vi "Get Mecanum Wheel Information.vi"(8 "error in (no error)":errorcluster, 11 "wheel in":refnum<class "NI_Robotics_Wheel.lvclass">) -> (0 "error out":errorcluster, 1 "wheel name":string, 2 "wheel parameters":T1={"wheel radius"=1.0, "gear ratio"=1.0, "forward rotation direction"=0} {"forward rotation direction" items=["Clockwise", "Counterclockwise"]}, 3 "wheel out":refnum<class "NI_Robotics_Wheel.lvclass">, 4 "motor communication":refnum<class "NI_Robotics_Motor Communication.lvclass">, 5 "roller orientation":T3 items=["Left", "Right"])   [LabVIEW 2017, in "NI_Robotics_Wheel.lvclass"]
doc: "Returns information, such as <B>wheel radius</B> and <B>gear ratio</B>, for the wheel you specify. You must manually select the polymorphic instance to use."
uses:
  <vilib>/robotics/Steering/Wheel/NI_Robotics_Wheel.lvclass
  <vilib>/robotics/Steering/Mecanum Wheel/Roller Orientation.ctl
  <vilib>/robotics/Steering/Wheel/Wheel Parameters.ctl
  <vilib>/robotics/Steering/Wheel/Rotation Direction.ctl
  <vilib>/robotics/Actuation/Motor Communication/NI_Robotics_Motor Communication.lvclass
  <vilib>/robotics/Steering/Mecanum Wheel/NI_Robotics_Mecanum Wheel.lvclass
  c:/Program Files (x86)/National Instruments/LabVIEW 2017/vi.lib/robotics/Steering/Wheel/NI_Robotics_Wheel.lvclass
  <vilib>/robotics/Steering/Wheel/NI_Robotics_Wheel.lvclass/NI_Robotics_Wheel.ctl
  <vilib>/robotics/Steering/Mecanum Wheel/NI_Robotics_Mecanum Wheel.lvclass/NI_Robotics_Mecanum Wheel.ctl
  <vilib>/robotics/Steering/Wheel/Get Motor Communication.vi
  <vilib>/robotics/Steering/Wheel/Get Wheel Parameters.vi
  <vilib>/robotics/Utilities/Generate Error.vi
  <vilib>/robotics/Utilities/Clear Specific Error.vi
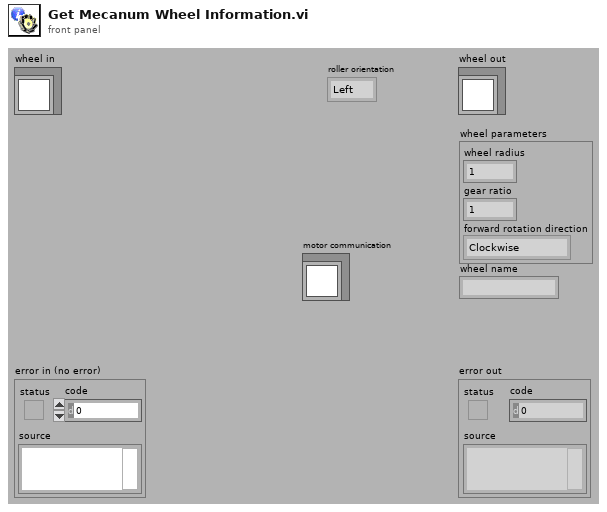
[diagram p1: front panel]
types:
  T1 = typedef "NI_Robotics_Wheel.lvclass/Wheel Parameters.ctl" = cluster{"wheel radius":dbl, "gear ratio":dbl, "forward rotation direction":T2}
  T2 = typedef "NI_Robotics_Wheel.lvclass/Rotation Direction.ctl" = u16
  T3 = typedef "NI_Robotics_Mecanum Wheel.lvclass/Roller Orientation.ctl" = u16
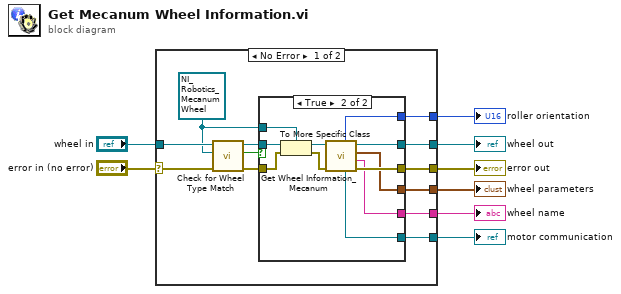
[diagram p0: block diagram]
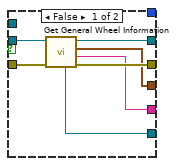
[diagram p2: hidden frame]
diagram:
  n1 = case shown="No Error" "error in (no error)" {
    selector: "error in (no error)" -> [w13 w40]
    tunnel: [w19 w40] -> w7
    tunnel: [w20 w39] -> w5
    tunnel: "wheel in" -> [w14 w39]
    tunnel: [w18 _] -> w4
    tunnel: [w17 _] -> w3
    tunnel: [w16 _] -> w2
    tunnel: [w15 _] -> w1
    frame No Error {
      w9 = refnum<class "NI_Robotics_Mecanum Wheel.lvclass"> refnum ("mecanum wheel in")
      n2 = call <vilib>:"Check for Wheel Type Match.vi"("error in (no error)"=w13, "target wheel type"=w9, "wheel in"=w14) -> ("error out"=w12:errorcluster, "match?"=w11:bool, "wheel out"=w10:refnum<class "NI_Robotics_Wheel.lvclass">)  [unwired: 6 in]
      n3 = case shown="True" w11 {
        tunnel: w10 -> [w27 w32]
        tunnel: [w24 w38] -> w20
        tunnel: [w25 w37] -> w19
        tunnel: [_ w36] -> w18
        tunnel: [w23 w35] -> w17
        tunnel: [w22 w34] -> w16
        tunnel: [w21 w33] -> w15
        tunnel: w9 -> [_ w30]
        tunnel: w12 -> [w26 w29]
        frame False {
          n4 = call <vilib>:"Get General Wheel Information.vi"("error in (no error)"=w26, "wheel in"=w27) -> ("error out"=w25:errorcluster, "wheel name"=w22:string, "wheel parameters"=w23:T1, "wheel out"=w24:refnum<class "NI_Robotics_Wheel.lvclass">, "motor communication"=w21:refnum<class "NI_Robotics_Motor Communication.lvclass">)  [unwired: 5 in]
        }
        frame True {
          n5 = To More Specific Class(target class=w30, reference=w32, error in=w29) -> (specific class reference=w31:refnum<class "NI_Robotics_Mecanum Wheel.lvclass">, error out=w28:errorcluster)
          n6 = call <vilib>:"Get Wheel Information_Mecanum.vi"("error in (no error)"=w28, "mecanum wheel in"=w31) -> ("error out"=w37:errorcluster, "wheel name"=w34:string, "wheel parameters"=w35:T1, "mecanum wheel out"=w38:refnum<class "NI_Robotics_Mecanum Wheel.lvclass">, "motor communication"=w33:refnum<class "NI_Robotics_Motor Communication.lvclass">, "roller orientation"=w36:T3)  [unwired: 4 in]
        }
      }
    }
    frame Error {
    }
  }
  "error out" <- w7
  "wheel out" <- w5
  "roller orientation" <- w4
  "wheel parameters" <- w3
  "wheel name" <- w2
  "motor communication" <- w1
